vi "TEST_bench_FXP_L_ye_Bend_u_singleAxis.vi"(6 "NS + 1":u8=9, 8 "Ldist":fxp<+/-,32,5>[](array[numeric])=[0.0, 0.0, 0.0, 0.0, 0.0, 0.0, 0.0, 0.0, 0.0, 0.0, 0.0, 0.0, 0.0, 0.0, 0.0, 0.0, 0.0, 0.0, 0.0, 0.0, 0.0, 0.0, 0.0, 0.0, 0.0, 0.0, 0.0, 0.0, 0.0, 0.0, 0.0, 0.0, 0.0, 0.0, 0.0, 0.0, 0.0, 0.0, 0.0, 0.0, 0.0, 0.0, 0.0, 0.0, 0.0, 0.0, 0.0, 0.0, 0.0, 0.0], 11 "x":fxp<+/-,32,5>[](array[numeric])=[0.0, 0.0, 0.0, 0.0, 0.0, 0.0, 0.0, 0.0, 0.0, 0.0, 0.0, 0.0, 0.0, 0.0, 0.0, 0.0, 0.0, 0.0, 0.0, 0.0, 0.0, 0.0, 0.0, 0.0, 0.0, 0.0, 0.0, 0.0, 0.0, 0.0, 0.0, 0.0, 0.0, 0.0, 0.0, 0.0, 0.0, 0.0, 0.0, 0.0, 0.0, 0.0, 0.0, 0.0, 0.0, 0.0, 0.0, 0.0, 0.0, 0.0]) -> ()   [LabVIEW 2017]
uses:
  fixed-point/typeDefs/x_vec_bram.ctl
  fixed-point/typeDefs/Lz_bram.ctl
  fixed-point/typeDefs/Bz_bram.ctl
  <vilib>/rvi/DataTransferAndStorage/Container/Common/niFpgaContainerExecOnDevCompGetState.vi
  <vilib>/rvi/Emulation/niFpgaEmulationIsFPGAContextNoSignature.vi
  <vilib>/rvi/DataTransferAndStorage/Container/Common/niFpgaContainerGetUniqueNameForEmu.vi
  <vilib>/rvi/Emulation/niFpgaProcessEmulError.vi
  <vilib>/rvi/Emulation/niFpgaSctlEmulationGetInTimedLoop.vi
  <vilib>/rvi/errors/nirviReportUnexpectedCaseInternalError (U32).vi
  <vilib>/rvi/Memory/Memory_Emulation/niFpgaMemoryEmulationCacheClearOnFirstRun.vi
  <vilib>/rvi/Memory/Memory_Emulation/nirvimemoryEmulationManagerCache_MakeExclusive.vi
  <vilib>/rvi/Memory/Memory_Emulation/niFpgaMemoryEmulationValidateCache.vi
  <vilib>/rvi/Memory/Memory_Emulation/nirvimemoryEmulationManagerCache_InsertValue.vi
  <vilib>/Utility/error.llb/Clear Errors.vi
  <vilib>/rvi/Memory/Memory_Emulation/nirvimemoryEmulationManagerCache_ReleaseExclusive.vi
  <vilib>/rvi/Memory/Memory_Emulation/nirvimemoryEmulationManagerCache_GetValue.vi
  <vilib>/rvi/Memory/Memory_Emulation/nirvimemoryEmulationManagerCache_SetValue.vi
  <vilib>/rvi/Emulation/niFpgaSctlEmulationResourceMgr.vi
  <vilib>/rvi/DataTransferAndStorage/Container/XNode/niFpgaContainer.xnode
  <vilib>/rvi/Memory/Memory_Emulation/niFpgaMemoryEmulationRefIn.vi
panel:
  in  "x_u(k)":fxp<+/-,32,8>
  out "xk_1_2":fxp<+/-,32,5>[](array[numeric])
  out "xk_1_1":fxp<+/-,32,5>[](array[numeric])
  in  "U(k): ux":fxp<+/-,18,5>
  in  "y(k)":fxp<+/-,18,5>
  out "yd_est":fxp<+/-,32,5>
  in  "Bz":fxp<+/-,32,5>[](array[numeric])=[0.0, 0.0, 0.0, 0.0, 0.0, 0.0, 0.0, 0.0, 0.0, 0.0, 0.0, 0.0, 0.0, 0.0, 0.0, 0.0, 0.0, 0.0, 0.0, 0.0, 0.0, 0.0, 0.0, 0.0, 0.0, 0.0, 0.0, 0.0, 0.0, 0.0, 0.0, 0.0, 0.0, 0.0, 0.0, 0.0, 0.0, 0.0, 0.0, 0.0, 0.0, 0.0, 0.0, 0.0, 0.0, 0.0, 0.0, 0.0, 0.0, 0.0]
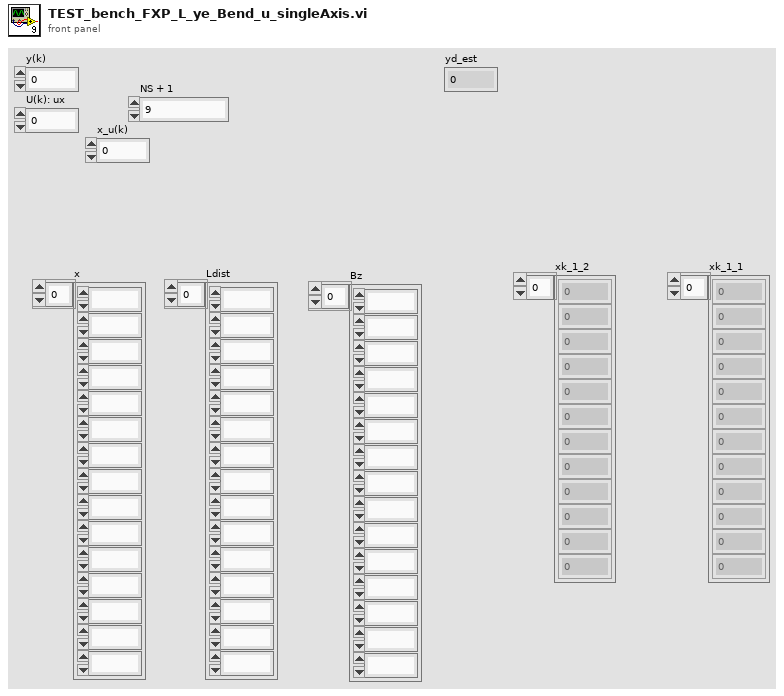
[diagram p1: front panel]
types:
  T1 = typedef "x_vec_bram.ctl" = refnum<k21>
  T2 = typedef "Bz_bram.ctl" = refnum<k21>
  T3 = typedef "Lz_bram.ctl" = refnum<k21>
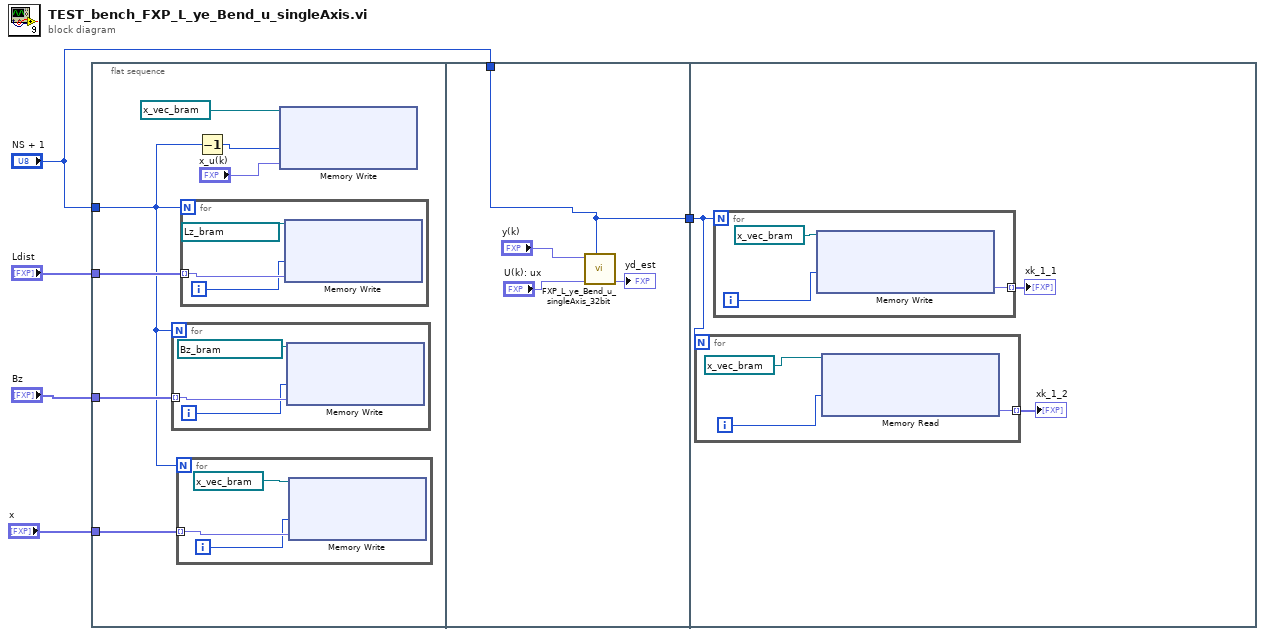
[diagram p0: block diagram]
diagram:
  n1 = flat-sequence {
    tunnel: "NS + 1" -> [w7]
    tunnel: "Ldist" -> [w12]
    tunnel: "x" -> [w11]
    tunnel: "Bz" -> [w10]
    tunnel: "NS + 1" -> [w22]
    tunnel: [w22] -> w1
    tunnel: w1 -> [w26]
    frame #0 {
      n2 = for {
        N: w7 -> [_]
        tunnel: w10 -> [w18] mode=indexing
        i -> [w17]
        n3 = xnode "Memory Write"("Address"=w17, "Data"=w18, "Memory In"=T2 "Bz_FXP_col1" ("Memory")) -> ()  [unwired: 1 out]
      }
      n4 = for {
        N: w7 -> [_]
        tunnel: w11 -> [w15] mode=indexing
        i -> [w14]
        n5 = xnode "Memory Write"("Address"=w14, "Data"=w15, "Memory In"=T1 "xk_1_0" ("Memory")) -> ()  [unwired: 1 out]
      }
      n6 = for {
        N: w7 -> [_]
        tunnel: w12 -> [w21] mode=indexing
        i -> [w20]
        n7 = xnode "Memory Write"("Address"=w20, "Data"=w21, "Memory In"=T3 "L_FXP_col1" ("Memory")) -> ()  [unwired: 1 out]
      }
      n8 = Decrement(x=w7) -> (x-1=w8:u8)
      n9 = xnode "Memory Write"("Address"=w8, "Data"="x_u(k)", "Memory In"=T1 "xk_1_2" ("Memory")) -> ()  [unwired: 1 out]
    }
    frame #1 {
      n10 = call "FXP_L_ye_Bend_u_singleAxis_32bit.vi"("NS"=w22, "U(k): ux"="U(k): ux", "Y(k): x"="y(k)") -> ("yd_est"=→"yd_est":fxp<+/-,32,5>)  [unwired: 6 in, 2 out]
    }
    frame #2 {
      n11 = for {
        N: w26 -> [_]
        tunnel: [w29] -> w27 mode=indexing
        i -> [w30]
        n12 = xnode "Memory Read"("Address"=w30, "Memory In"=T1 "xk_1_2" ("Memory")) -> ("Data"=w29:fxp<+/-,32,6>)  [unwired: 1 out]
      }
      "xk_1_2" <- w27
      n13 = for {
        N: w26 -> [_]
        tunnel: [w33] -> w28 mode=indexing
        i -> [w34]
        n14 = xnode "Memory Write"("Address"=w34, "Memory In"=T1 "xk_1_1" ("Memory")) -> ("Data"=w33:fxp<+/-,32,6>)  [unwired: 1 out]
      }
      "xk_1_1" <- w28
    }
  }
